vi "help.vi"() -> (3 "Cancelled?":bool)   [LabVIEW 2012]
doc: "Use this template to create a dialog box with event handling."
panel:
  in  "OK":bool
  # "Instruções básicas para usar o programa IxV\n\nO programa irá salvar um arquivo com os dados da medição no local que o usuário escolher no campo Local do Arquivo\n\nO usuário pode escolher entre os dois formatos de arquivo, .txt ou .csv(abre como planilha no excel).\n\nO campo N° medições por ponto são o número de vezes que o mesmo ponto da curva será medido. A média será feita e plotada no gráfico, assim como o desvio padrão. Ou seja, quantos mais medidas por ponto, melhor será a curva, porém o tempo por medição será maior.\n\nO campo N° curvas são o número de medições e curvas serão geradas com os parâmetros determinados.\n\nO usuário poderá controlar o número de pontos antes e no joelho da curva, assim como a tensão máxima e a tensão no joelho.\n\nA caixa de seleção Print da curva(s), ao selecionada, irá tirar uma Screenshot da tela do programa ao final de cada curva gerada, e serão salvas no mesmo diretório escolhido para o arquivo dos dados da medição. O botão Start inicia a medição.\n\nAo iniciar a medição você porderá ver a curva sendo gerada em tempo real. Se o usuário não estiver satisfeito, podera parar e medição no meio e voltar para a tela de Entrada de dados. Obs: o usuário só poderá voltar se a medição estiver parada ou finalizada.\n\nPara mostrar o desvio padrão, caso exista, basta clicar com o botoão direito na opção de desvio do gráfico e selecionar plot visible.\n\n                                                                                 Outras opções como corrigir curva ainda não foram implementadas"
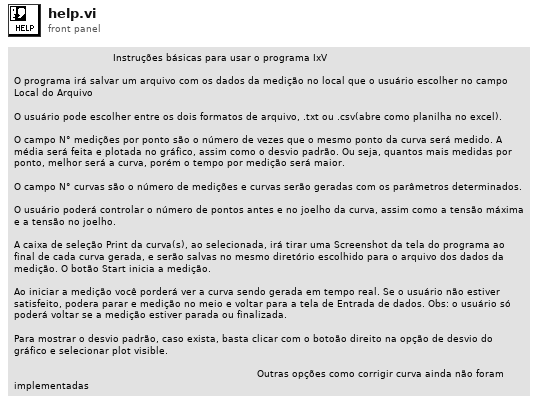
[diagram p1: front panel]
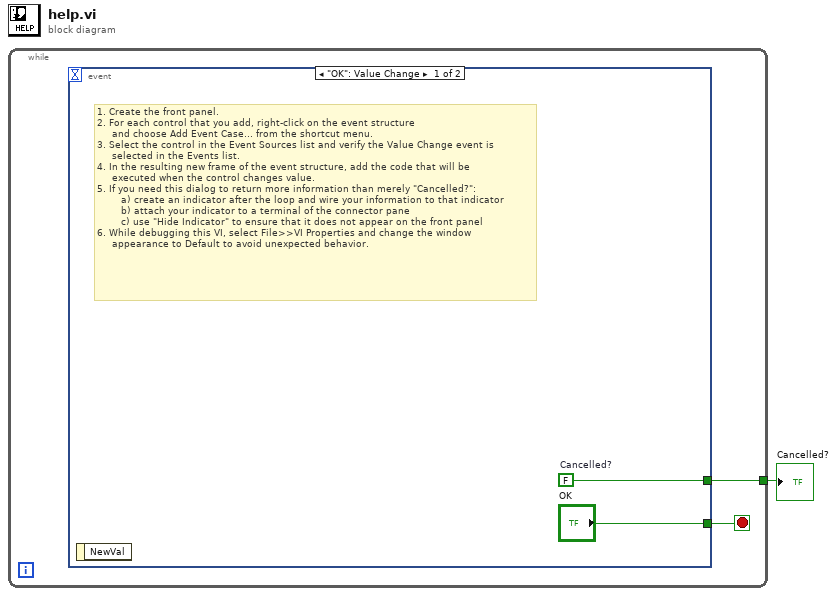
[diagram p0: block diagram]
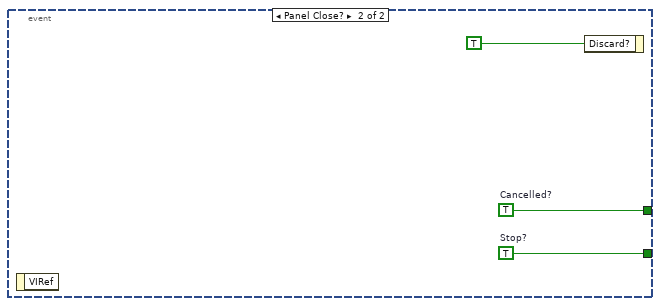
[diagram p2: hidden frame]
diagram:
  n1 = while {
    tunnel: [w2] -> w1
    stop <- w3 stop-if-true
    n2 = event shown="[0] \"OK\": Value Change" {
      selector: _ -> [_ _]
      dyn-events: _ -> [_ _]
      timeout: _ -> [_ _]
      tunnel: ["OK" w7] -> w3
      tunnel: [w5 w6] -> w2
      event "OK": Value Change {
        w5 = FALSE  # Cancelled?
        # "1. Create the front panel.\n2. For each control that you add, right-click on the event structure \n     and choose Add Event Case... from the shortcut menu.\n3. Select the control in the Event Sources list and verify the Value Change event is \n     selected in the Events list.\n4. In the resulting new frame of the event structure, add the code that will be \n     executed when the control changes value.\n5. If you need this dialog to return more information than merely \"Cancelled?\":\n        a) create an indicator after the loop and wire your information to that indicator\n        b) attach your indicator to a terminal of the connector pane\n        c) use \"Hide Indicator\" to ensure that it does not appear on the front panel\n6. While debugging this VI, select File>>VI Properties and change the window \n     appearance to Default to avoid unexpected behavior."
        n3 = event-data() -> ()  [unwired: 1 in, 1 out]
      }
      event Panel Close? {
        w6 = TRUE  # Cancelled?
        w7 = TRUE  # Stop?
        n4 = event-data() -> ()  [unwired: 1 in, 1 out]
        n5 = event-data("Discard?"=TRUE) -> ()  [unwired: 1 in, 1 out]
      }
    }
  }
  "Cancelled?" <- w1
